vi "Serve File.vi"(5 "Response":refnum<class "Response.lvclass">, 7 "Request":refnum<class "Request.lvclass">, 8 "error in (no error)":errorcluster) -> (0 "error out":errorcluster, 2 "Handled?":bool)   [LabVIEW 2023, in "Server.lvclass"]
uses:
  Server.lvclass
  Request/Request.lvclass
  Response/Response.lvclass
  Request/Get Request.vi
  Server.lvclass/Server.ctl
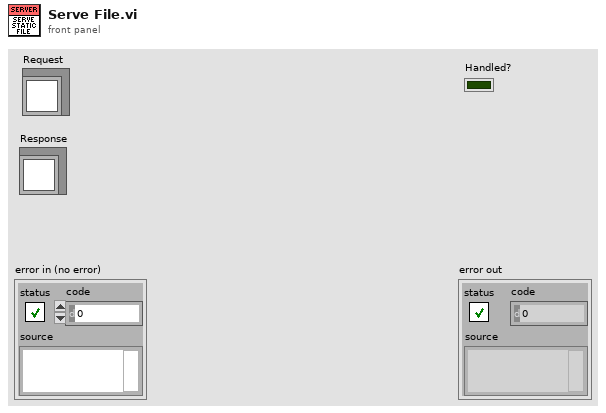
[diagram p1: front panel]
types:
  T1 = typedef "Server.lvclass/ObjectAttributes.ctl" = cluster{"Static Data":path, "MIME Types":variant, "Shutdown":bool, "API Queue":refnum<queue>}
  T2 = typedef "Request.ctl" = cluster{"Method":string, "URI":string, "Protocol":string, "Raw Path":string, "Query":string, "Fragment":string, "Raw Body":string, "Headers":variant, "Parameters":variant, "Body":variant, "Raw Header":string, "Path":string[]}
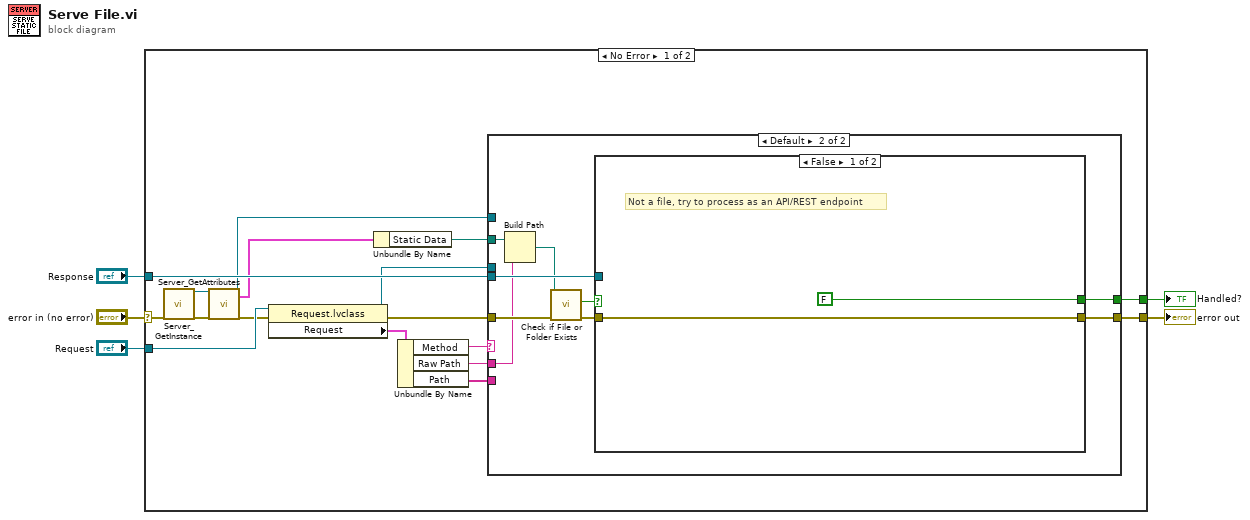
[diagram p0: block diagram]
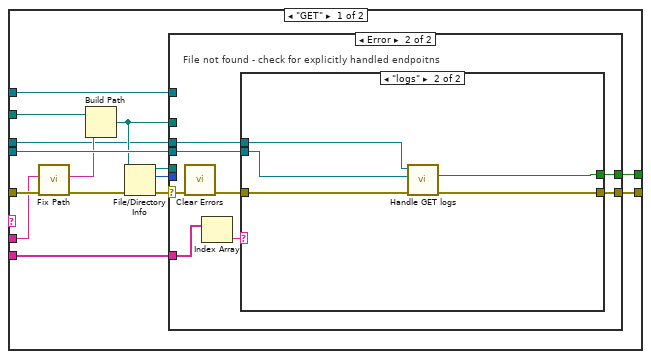
[diagram p2: hidden frame]
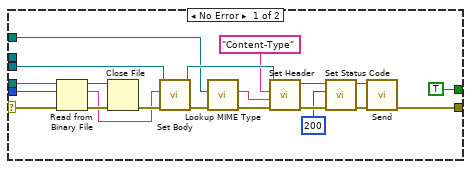
[diagram p3: hidden frame]
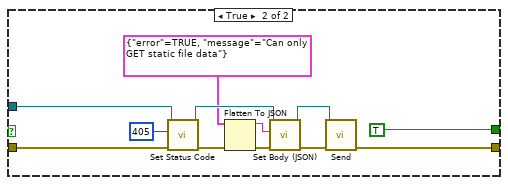
[diagram p5: hidden frame]
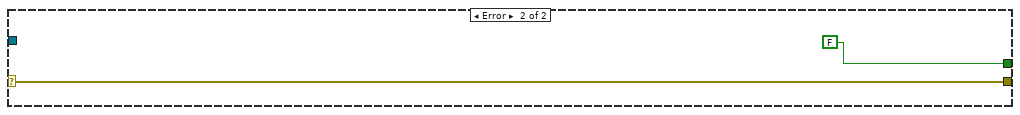
[diagram p6: hidden frame]
diagram:
  n1 = case shown="No Error" "error in (no error)" {
    selector: "error in (no error)" -> [w14 w97]
    tunnel: [w18 w97] -> w4
    tunnel: "Request" -> [w22 _]
    tunnel: "Response" -> [w17 _]
    tunnel: [w15 FALSE] -> w1
    frame No Error {
      n2 = call "Server_GetInstance.vi"("error in (no error)"=w14) -> ("reference out"=w9:refnum<class "Server.lvclass">, "error out"=w10:errorcluster)  [unwired: 14 in, 3 out]
      n3 = call "Server_GetAttributes.vi"("reference in"=w9, "error in (no error)"=w10) -> ("reference out"=w8:refnum<class "Server.lvclass">, "Data"=w12:T1, "error out"=w13:errorcluster)  [unwired: 14 in, 1 out]
      n4 = property class="Request.lvclass"(reference=w22, error in=w13) -> (reference out=w6:refnum<class "Request.lvclass">, error out=w19:errorcluster, "Request"=w21:T2)
      n5 = Unbundle By Name(w12) -> ("Static Data"=w11:path)
      n6 = Unbundle By Name(w21) -> ("Method"=w20:string, "Raw Path"=w16:string, "Path"=w7:string[])
      n7 = case shown="Default" w20 {
        tunnel: w19 -> [w30 w81]
        tunnel: [w34 w80] -> w18
        tunnel: w17 -> [w33 w79]
        tunnel: w16 -> [w28 w76]
        tunnel: w11 -> [w37 w77]
        tunnel: w8 -> [w25 _]
        tunnel: [w26 w78] -> w15
        tunnel: w7 -> [w24 _]
        tunnel: w6 -> [w23 _]
        frame "GET" {
          n8 = call "Fix Path.vi"("error in (no error)"=w30, "Request Path"=w28) -> ("error out"=w29:errorcluster, "Fixed"=w27:string)  [unwired: 8 in]
          n9 = Build Path(base path=w37, name or relative path=w27) -> (appended path=w32:path)
          n10 = File/Directory Info(path=w32, error in=w29) -> (path out=w35:path, size=w31:i64, error out=w36:errorcluster)  [unwired: 4 out]
          n11 = case shown="Error" w36 {
            selector: w36 -> [w58 w65]
            tunnel: w35 -> [w57 _]
            tunnel: [w51 w63] -> w34
            tunnel: w33 -> [w52 w59]
            tunnel: w32 -> [w45 _]
            tunnel: w25 -> [_ _]
            tunnel: w31 -> [w43 _]
            tunnel: [TRUE w66] -> w26
            tunnel: w24 -> [_ w62]
            tunnel: w23 -> [_ w60]
            frame No Error {
              n12 = Read from Binary File(8:w58, 10:w43, 11:w57) -> (0:w56:errorcluster, 2:w53:string, 3:w55:refnum<file>)  [unwired: 3 in, 1 out]
              n13 = Close File(refnum=w55, error in=w56) -> (error out=w54:errorcluster)  [unwired: 1 out]
              n14 = call "Set Body.vi"("error in (no error)"=w54, "Body"=w53, "Response in"=w52) -> ("error out"=w47:errorcluster, "Response out"=w49:refnum<class "Response.lvclass">)  [unwired: 7 in]
              n15 = call "Lookup MIME Type.vi"("error in (no error)"=w47, "Path"=w45) -> ("error out"=w46:errorcluster, "MIME Type"=w44:string)  [unwired: 8 in]
              n16 = call "Set Header.vi"("error in (no error)"=w46, "Value"=w44, "Header"="Content-Type", "Response in"=w49) -> ("error out"=w50:errorcluster, "Response out"=w41:refnum<class "Response.lvclass">)  [unwired: 5 in, 1 out]
              n17 = call "Set Status Code.vi"("error in (no error)"=w50, "Status Code"=u16 200, "Response in"=w41) -> ("error out"=w42:errorcluster, "Response out"=w40:refnum<class "Response.lvclass">)  [unwired: 7 in]
              n18 = call "Send.vi"("error in (no error)"=w42, "Response in"=w40) -> ("error out"=w51:errorcluster)  [unwired: 9 in]
            }
            frame Error {
              # "File not found - check for explicitly handled endpoitns"
              n19 = call <vilib>:"Clear Errors.vi"("error in (no error)"=w65) -> ("error out"=w64:errorcluster)  [unwired: 5 in, 1 out]
              n20 = Index Array(array=w62) -> (element=w61:string)  [unwired: 1 in]
              n21 = case shown="\"logs\"" w61 {
                tunnel: [_ w68] -> w66
                tunnel: w64 -> [w67 w72]
                tunnel: [w67 w71] -> w63
                tunnel: w60 -> [_ w70]
                tunnel: w59 -> [_ w69]
                frame Default {
                }
                frame "logs" {
                  n22 = call "Handle GET logs.vi"("error in (no error)"=w72, "Response"=w69, "Request in"=w70) -> ("error out"=w71:errorcluster, "Handled?"=w68:bool)  [unwired: 7 in]
                }
              }
            }
          }
        }
        frame Default {
          n23 = Build Path(base path=w77, name or relative path=w76) -> (appended path=w74:path)
          n24 = call <vilib>:"Check if File or Folder Exists.vi"("error in (no error)"=w81, "path"=w74) -> ("error out"=w75:errorcluster, "file or folder exists?"=w73:bool)  [unwired: 7 in, 1 out]
          n25 = case shown="False" w73 {
            tunnel: w75 -> [w83 w88]
            tunnel: [w83 w87] -> w80
            tunnel: w79 -> [_ w86]
            tunnel: [FALSE TRUE] -> w78
            frame False {
              # "Not a file, try to process as an API/REST endpoint"
            }
            frame True {
              n26 = call "Set Status Code.vi"("error in (no error)"=w88, "Status Code"=u16 405, "Response in"=w86) -> ("error out"=w95:errorcluster, "Response out"=w91:refnum<class "Response.lvclass">)  [unwired: 7 in]
              n27 = Flatten To JSON(anything=cluster{"error":bool, "message":string} {"error"=TRUE, "message"="Can only GET static file data"}, error in (no error)=w95) -> (JSON string=w89:string, 11:w93:errorcluster)  [unwired: 1 in]
              n28 = call "Set Body (JSON).vi"("error in (no error)"=w93, "Body (as JSON)"=w89, "Response in"=w91) -> ("error out"=w92:errorcluster, "Response out"=w90:refnum<class "Response.lvclass">)  [unwired: 7 in]
              n29 = call "Send.vi"("error in (no error)"=w92, "Response in"=w90) -> ("error out"=w87:errorcluster)  [unwired: 9 in]
            }
          }
        }
      }
    }
    frame Error {
    }
  }
  "error out" <- w4
  "Handled?" <- w1
